vi "Start.vi"(8 "error in (no error)":errorcluster, 11 "XNET Base CFG in":refnum<class "XNET Base CFG.lvclass">) -> (0 "error out":errorcluster, 3 "XNET Base CFG out":refnum<class "XNET Base CFG.lvclass">)   [LabVIEW 2023, in "XNET Base CFG.lvclass"]
doc: "Starts communication for the specified XNET session."
uses:
  XNET Base CFG.lvclass
  XNET Base CFG.lvclass/XNET Base CFG.ctl
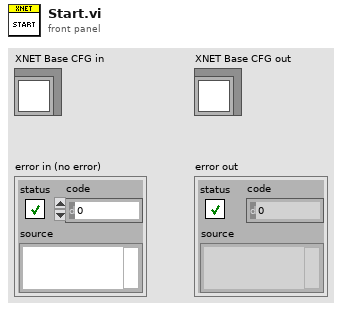
[diagram p1: front panel]
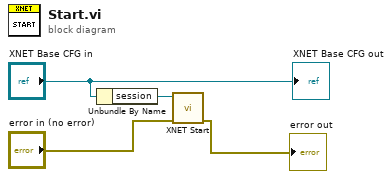
[diagram p0: block diagram]
diagram:
  n1 = Unbundle By Name("XNET Base CFG in") -> ("session"=w4:refnum<k21>)
  n2 = call <vilib>:"XNET Start.vi"("session in"=w4, "error in (no error)"="error in (no error)") -> ("error out"=→"error out":errorcluster)  [unwired: 12 in, 1 out]
  "XNET Base CFG out" <- "XNET Base CFG in"
